vi "Hadamard vs DAQ.vi"() -> ()   [LabVIEW 2023]
uses:
  <vilib>/Utility/miscctls.llb/LVBoundsTypeDef.ctl
  <vilib>/Utility/miscctls.llb/LVRectTypeDef.ctl
panel:
  in  "Plot Area:Size":T1
  out "?":errorcluster
  in  "error in (no error)":errorcluster
  in  "Z Scale.Marker Values[]":cluster{dbl, u32}[](array[cluster])=[{0.0, 0}, {100.0, 16777215}]
  out "Delay":i32=20
  out "Intensity Graph":dbl[][](graph)=[[0.0, 1.0, 0.0, 1.0, 1.0, 0.0, 1.0, 0.0, 0.0, 1.0, 0.0, 1.0, 1.0, 0.0, 1.0, 0.0], [0.0, 1.0, 0.0, 1.0, 1.0, 0.0, 1.0, 0.0, 0.0, 1.0, 0.0, 1.0, 1.0, 0.0, 1.0, 0.0], [1.0, 0.0, 1.0, 0.0, 0.0, 1.0, 0.0, 1.0, 1.0, 0.0, 1.0, 0.0, 0.0, 1.0, 0.0, 1.0], [1.0, 0.0, 1.0, 0.0, 0.0, 1.0, 0.0, 1.0, 1.0, 0.0, 1.0, 0.0, 0.0, 1.0, 0.0, 1.0], [0.0, 1.0, 0.0, 1.0, 1.0, 0.0, 1.0, 0.0, 0.0, 1.0, 0.0, 1.0, 1.0, 0.0, 1.0, 0.0], [0.0, 1.0, 0.0, 1.0, 1.0, 0.0, 1.0, 0.0, 0.0, 1.0, 0.0, 1.0, 1.0, 0.0, 1.0, 0.0], [1.0, 0.0, 1.0, 0.0, 0.0, 1.0, 0.0, 1.0, 1.0, 0.0, 1.0, 0.0, 0.0, 1.0, 0.0, 1.0], [1.0, 0.0, 1.0, 0.0, 0.0, 1.0, 0.0, 1.0, 1.0, 0.0, 1.0, 0.0, 0.0, 1.0, 0.0, 1.0], [0.0, 1.0, 0.0, 1.0, 1.0, 0.0, 1.0, 0.0, 0.0, 1.0, 0.0, 1.0, 1.0, 0.0, 1.0, 0.0], [0.0, 1.0, 0.0, 1.0, 1.0, 0.0, 1.0, 0.0, 0.0, 1.0, 0.0, 1.0, 1.0, 0.0, 1.0, 0.0], [1.0, 0.0, 1.0, 0.0, 0.0, 1.0, 0.0, 1.0, 1.0, 0.0, 1.0, 0.0, 0.0, 1.0, 0.0, 1.0], [1.0, 0.0, 1.0, 0.0, 0.0, 1.0, 0.0, 1.0, 1.0, 0.0, 1.0, 0.0, 0.0, 1.0, 0.0, 1.0], [0.0, 1.0, 0.0, 1.0, 1.0, 0.0, 1.0, 0.0, 0.0, 1.0, 0.0, 1.0, 1.0, 0.0, 1.0, 0.0], [0.0, 1.0, 0.0, 1.0, 1.0, 0.0, 1.0, 0.0, 0.0, 1.0, 0.0, 1.0, 1.0, 0.0, 1.0, 0.0], [1.0, 0.0, 1.0, 0.0, 0.0, 1.0, 0.0, 1.0, 1.0, 0.0, 1.0, 0.0, 0.0, 1.0, 0.0, 1.0], [1.0, 0.0, 1.0, 0.0, 0.0, 1.0, 0.0, 1.0, 1.0, 0.0, 1.0, 0.0, 0.0, 1.0, 0.0, 1.0]]
  out "N":i32=16
  in  "stop":bool
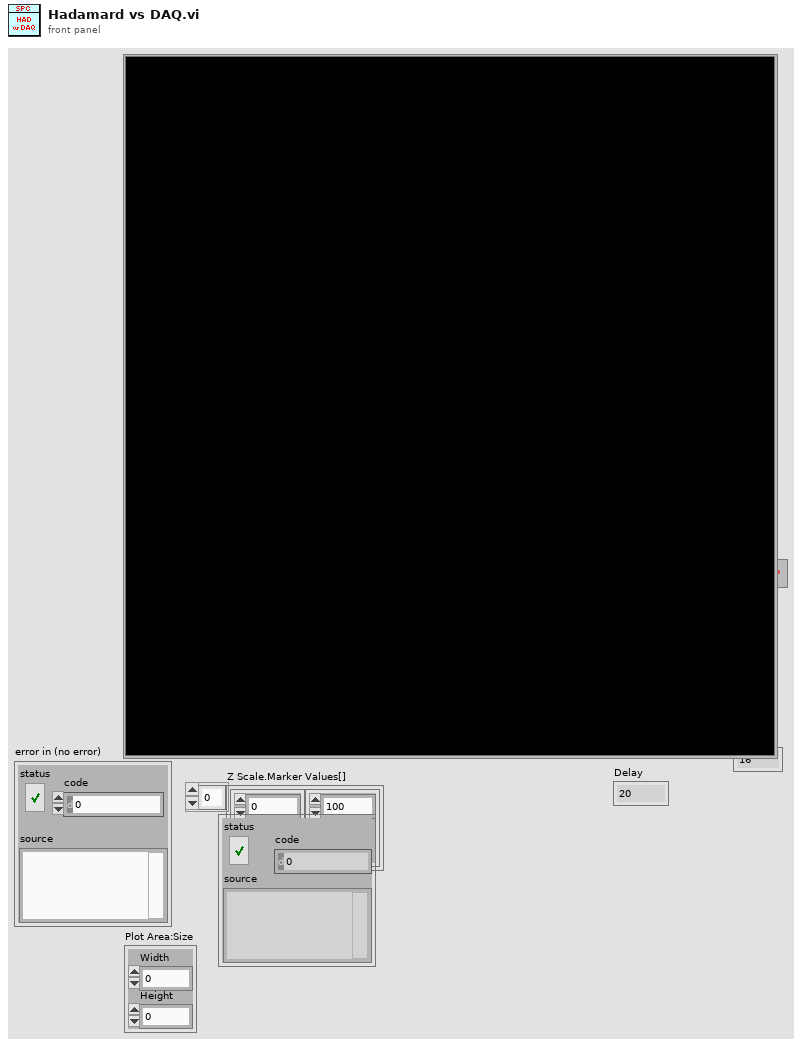
[diagram p1: front panel]
types:
  T1 = typedef "LVBoundsTypeDef.ctl" = cluster{"Width":u32, "Height":u32}
  T2 = typedef "LVRectTypeDef.ctl" = cluster{"Left":i16, "Top":i16, "Right":i16, "Bottom":i16}
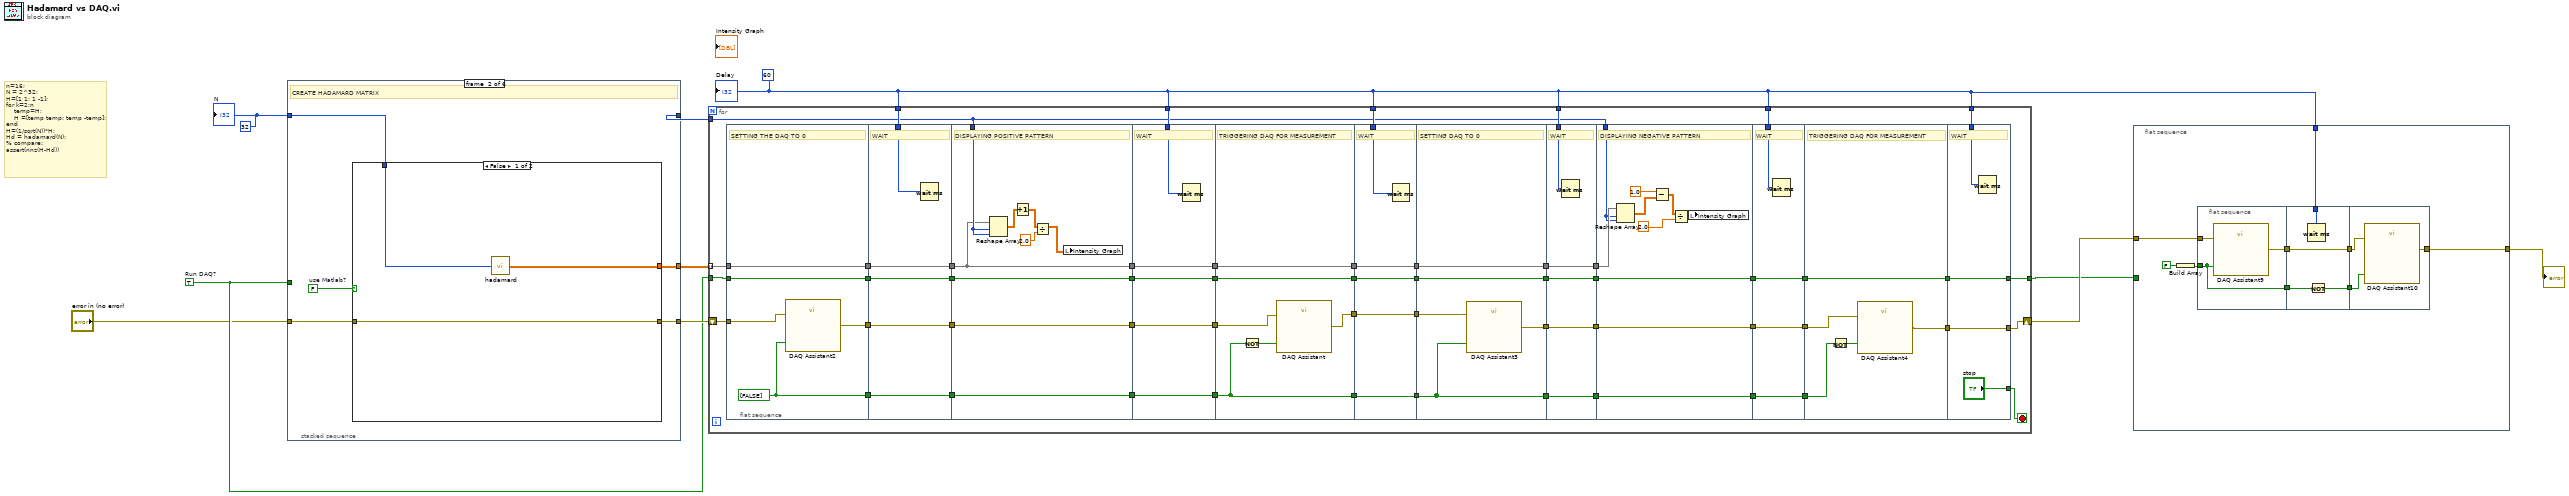
[diagram p0: block diagram]
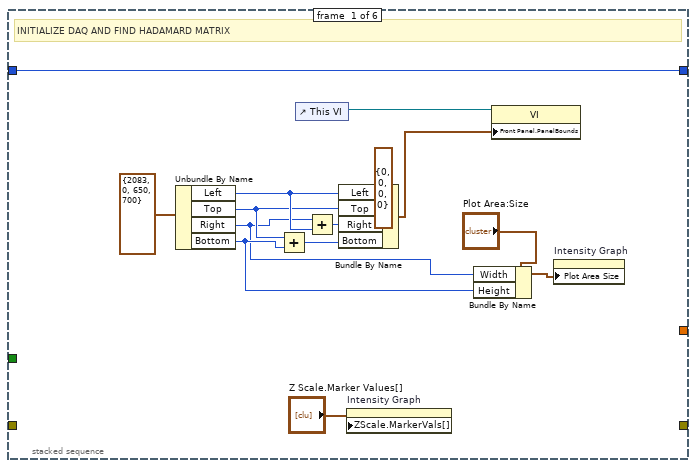
[diagram p2: hidden frame]
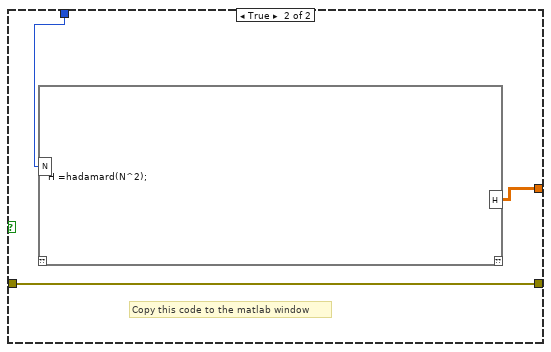
[diagram p3: hidden frame]
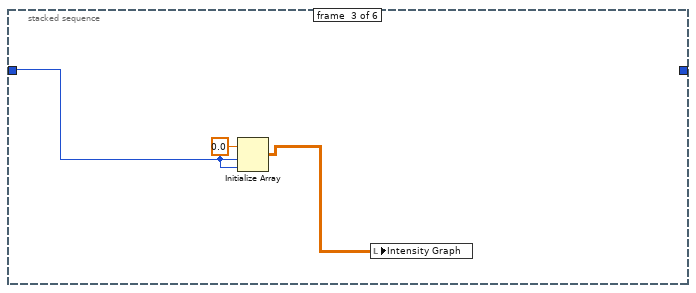
[diagram p4: hidden frame]
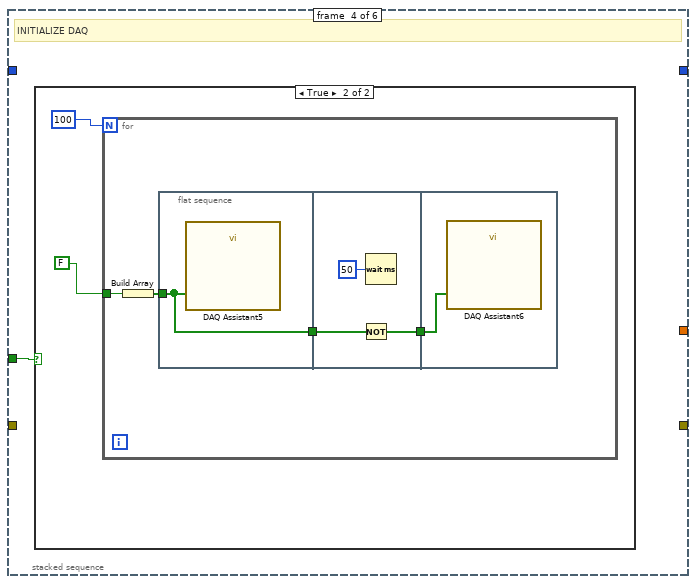
[diagram p5: hidden frame]
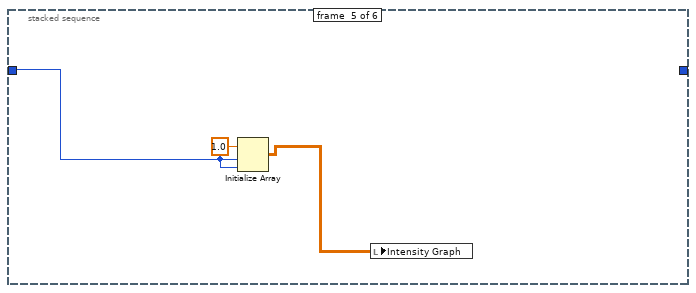
[diagram p7: hidden frame]
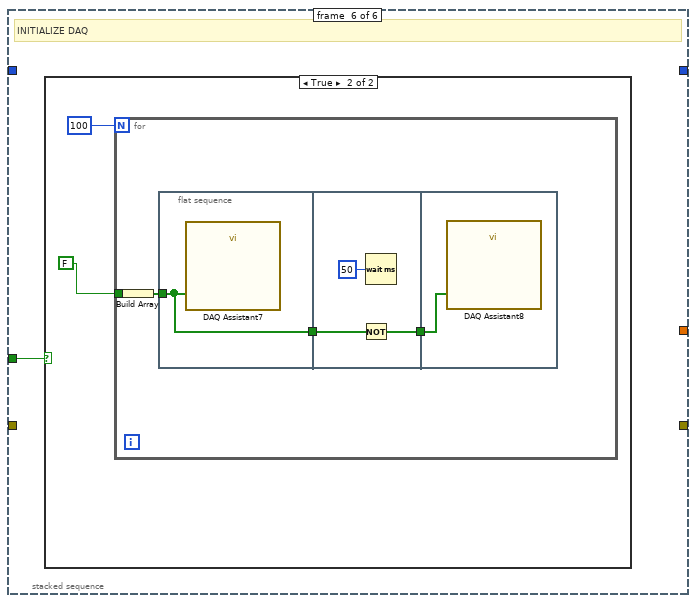
[diagram p8: hidden frame]
diagram:
  w4 = TRUE  # Run DAQ?
  w3 = 60 ("Delay")
  w7 = 32 ("N")
  # "n=16;\nN = 2^32;\nH=[1 1; 1 -1];\nfor k=2:n\n    temp=H;\n    H =[temp temp; temp -temp];\nend\nH=(1/sqrt(N))*H;\nHd = hadamard(N);\n% compare:\nassert(nnz(H-Hd))"
  n1 = stacked-sequence {
    tunnel: [_ w25 _ _ _ _] -> w9
    tunnel: w7 -> [w24 w28 w38 _ w53 _]
    tunnel: [w24 _ _ _ _ _] -> w8
    tunnel: [_ w27 _ _ _ _] -> w10
    tunnel: w4 -> [_ _ _ w39 _ w54]
    tunnel: "error in (no error)" -> [_ w26 _ _ _ _]
    frame #0 {
      # "INITIALIZE DAQ AND FIND HADAMARD MATRIX"
      n2 = Unbundle By Name(T2 {"Left"=2083, "Top"=0, "Right"=650, "Bottom"=700} ("Front Panel Window:Panel Bounds")) -> ("Left"=w20:i16, "Top"=w12:i16, "Right"=w11:i16, "Bottom"=w13:i16)
      n3 = Add(x=w12, y=w13) -> (x+y=w17:i16)
      n4 = control-ref of="This VI"() -> (w22:refnum<vi>)
      n5 = Add(x=w11, y=w20) -> (x+y=w19:i16)
      n6 = Bundle By Name(cluster=T2 {"Left"=0, "Top"=0, "Right"=0, "Bottom"=0} ("output cluster"), "Left"=w20, "Top"=w12, "Right"=w19, "Bottom"=w17) -> (w18:T2)
      n7 = property on="Intensity Graph" class="IntGraph (strict)"("ZScale.MarkerVals[]"="Z Scale.Marker Values[]") -> ()  [unwired: 2 in, 2 out]
      n8 = Bundle By Name(cluster="Plot Area:Size", "Width"=w11, "Height"=w13) -> (w14:T1)
      n9 = property class="VI"(reference=w22, "Front Panel.PanelBounds"=w18) -> ()  [unwired: 1 in, 2 out]
      n10 = property on="Intensity Graph" class="IntGraph (strict)"("Plot Area Size"=w14) -> ()  [unwired: 2 in, 2 out]
    }
    frame #1 {
      w29 = FALSE  # use Matlab?
      # "CREATE HADAMARD MATRIX"
      n11 = case shown="False" w29 {
        tunnel: w28 -> [w32 w34]
        tunnel: [w31 w33] -> w25
        tunnel: [w30 w35] -> w27
        tunnel: w26 -> [w30 w35]
        frame False {
          n12 = call "hadamard.vi"("N"=w32) -> ("Intensity Graph"=w31:dbl[][])
        }
        frame True {
          # "Copy this code to the matlab window"
          n13 = script code="H =hadamard(N^2);"("N"=w34) -> ("H"=w33:dbl[][])  [unwired: 1 in, 1 out]
        }
      }
    }
    frame #2 {
      n14 = Initialize Array(0.0 ("element"), w38, w38) -> (w37:dbl[][])
      n15 = local write "Intensity Graph"(w37) -> ()
    }
    frame #3 {
      # "INITIALIZE DAQ"
      n16 = case shown="True" w39 {
        frame False {
        }
        frame True {
          n17 = for {
            N: 100 -> [_]
            tunnel: FALSE -> [w44]
            n18 = Build Array(w44) -> (w45:bool[])
            n19 = flat-sequence {
              tunnel: w45 -> [w46]
              tunnel: [w46] -> w42
              tunnel: [w47] -> w43
              tunnel: w42 -> [w48]
              tunnel: w43 -> [w50]
              frame #0 {
                n20 = call "DAQ Assistant5"("data"=w46) -> ()  [unwired: 17 in, 2 out]
              }
              frame #1 {
                n21 = Not(x=w48) -> (.not. x?=w47:bool[])
                n22 = Wait (ms)(milliseconds to wait=u32 50) -> ()  [unwired: 1 out]
              }
              frame #2 {
                n23 = call "DAQ Assistant6"("data"=w50) -> ()  [unwired: 17 in, 2 out]
              }
            }
          }
        }
      }
    }
    frame #4 {
      n24 = Initialize Array(1.0 ("element"), w53, w53) -> (w52:dbl[][])
      n25 = local write "Intensity Graph"(w52) -> ()
    }
    frame #5 {
      # "INITIALIZE DAQ"
      n26 = case shown="True" w54 {
        frame False {
        }
        frame True {
          n27 = for {
            N: 100 -> [_]
            tunnel: FALSE -> [w59]
            n28 = Build Array(w59) -> (w60:bool[])
            n29 = flat-sequence {
              tunnel: w60 -> [w61]
              tunnel: [w61] -> w57
              tunnel: [w62] -> w58
              tunnel: w57 -> [w63]
              tunnel: w58 -> [w65]
              frame #0 {
                n30 = call "DAQ Assistant7"("data"=w61) -> ()  [unwired: 17 in, 2 out]
              }
              frame #1 {
                n31 = Not(x=w63) -> (.not. x?=w62:bool[])
                n32 = Wait (ms)(milliseconds to wait=u32 50) -> ()  [unwired: 1 out]
              }
              frame #2 {
                n33 = call "DAQ Assistant8"("data"=w65) -> ()  [unwired: 17 in, 2 out]
              }
            }
          }
        }
      }
    }
  }
  n34 = for {
    tunnel: w9 -> [w118] mode=indexing
    tunnel: w3 -> [w111]
    tunnel: w3 -> [w110]
    tunnel: w3 -> [w109]
    tunnel: w3 -> [w100]
    tunnel: w3 -> [w99]
    tunnel: w3 -> [w94]
    shift-right: [w92] -> w6
    shift-left: w10 -> [w80]
    tunnel: w8 -> [w79]
    tunnel: w4 -> [w78]
    tunnel: [w66] -> w2
    stop <- w93 stop-if-true
    n35 = flat-sequence {
      tunnel: w118 -> [w123]
      tunnel: [w123] -> w116
      tunnel: [w122] -> w112
      tunnel: [w121] -> w84
      tunnel: w80 -> [w120]
      tunnel: w78 -> [w119]
      tunnel: [w119] -> w74
      tunnel: [w128] -> w117
      tunnel: w116 -> [w128]
      tunnel: [w127] -> w113
      tunnel: w112 -> [w127]
      tunnel: w111 -> [w126]
      tunnel: w84 -> [w125]
      tunnel: [w125] -> w83
      tunnel: [w124] -> w75
      tunnel: w74 -> [w124]
      tunnel: w117 -> [w130]
      tunnel: w79 -> [w137]
      tunnel: [w136] -> w114
      tunnel: w113 -> [w136]
      tunnel: [w130] -> w106
      tunnel: w83 -> [w133]
      tunnel: [w133] -> w82
      tunnel: [w129] -> w76
      tunnel: w75 -> [w129]
      tunnel: [w142] -> w115
      tunnel: w114 -> [w142]
      tunnel: w110 -> [w141]
      tunnel: [w140] -> w107
      tunnel: w106 -> [w140]
      tunnel: w82 -> [w139]
      tunnel: [w139] -> w81
      tunnel: [w138] -> w77
      tunnel: w76 -> [w138]
      tunnel: w115 -> [w147]
      tunnel: [w148] -> w108
      tunnel: w107 -> [w148]
      tunnel: [w147] -> w103
      tunnel: [w146] -> w86
      tunnel: w81 -> [w145]
      tunnel: w77 -> [w144]
      tunnel: [w144] -> w72
      tunnel: w109 -> [w153]
      tunnel: [w152] -> w105
      tunnel: w108 -> [w152]
      tunnel: [w151] -> w104
      tunnel: w103 -> [w151]
      tunnel: w86 -> [w150]
      tunnel: [w150] -> w85
      tunnel: [w149] -> w73
      tunnel: w72 -> [w149]
      tunnel: w105 -> [w158]
      tunnel: [w158] -> w102
      tunnel: w104 -> [w157]
      tunnel: [w157] -> w95
      tunnel: [w156] -> w90
      tunnel: w85 -> [w155]
      tunnel: w73 -> [w154]
      tunnel: [w154] -> w67
      tunnel: w102 -> [w163]
      tunnel: [w163] -> w101
      tunnel: w100 -> [w162]
      tunnel: [w161] -> w96
      tunnel: w95 -> [w161]
      tunnel: w90 -> [w160]
      tunnel: [w160] -> w89
      tunnel: [w159] -> w68
      tunnel: w67 -> [w159]
      tunnel: w101 -> [w172]
      tunnel: w79 -> [w171]
      tunnel: [w169] -> w97
      tunnel: w96 -> [w169]
      tunnel: w89 -> [w168]
      tunnel: [w168] -> w88
      tunnel: [w164] -> w69
      tunnel: w68 -> [w164]
      tunnel: w99 -> [w177]
      tunnel: [w176] -> w98
      tunnel: w97 -> [w176]
      tunnel: w88 -> [w175]
      tunnel: [w175] -> w87
      tunnel: [w174] -> w70
      tunnel: w69 -> [w174]
      tunnel: w98 -> [w182]
      tunnel: [w181] -> w91
      tunnel: w87 -> [w178]
      tunnel: [w180] -> w71
      tunnel: w70 -> [w180]
      tunnel: w94 -> [w186]
      tunnel: ["stop"] -> w93
      tunnel: [w184] -> w92
      tunnel: w91 -> [w184]
      tunnel: [w183] -> w66
      tunnel: w71 -> [w183]
      frame #0 {
        w122 = bool[] [FALSE] ("data")
        # "SETTING THE DAQ TO 0"
        n36 = call "DAQ Assistant2"("data"=w122, "error in"=w120) -> ("error out"=w121:errorcluster)  [unwired: 16 in, 1 out]
      }
      frame #1 {
        # "WAIT"
        n37 = Wait (ms)(milliseconds to wait=w126) -> ()  [unwired: 1 out]
      }
      frame #2 {
        # "DISPLAYING POSITIVE PATTERN"
        n38 = Reshape Array(w130, w137, w137) -> (w132:dbl[][])
        n39 = Increment(x=w132) -> (x+1=w131:dbl[][])
        n40 = Divide(x=w131, y=2.0) -> (x/y=w134:dbl[][])
        n41 = local write "Intensity Graph"(w134) -> ()
      }
      frame #3 {
        # "WAIT"
        n42 = Wait (ms)(milliseconds to wait=w141) -> ()  [unwired: 1 out]
      }
      frame #4 {
        # "TRIGGERING DAQ FOR MEASUREMENT"
        n43 = Not(x=w147) -> (.not. x?=w143:bool[])
        n44 = call "DAQ Assistant"("data"=w143, "error in"=w145) -> ("error out"=w146:errorcluster)  [unwired: 16 in, 1 out]
      }
      frame #5 {
        # "WAIT"
        n45 = Wait (ms)(milliseconds to wait=w153) -> ()  [unwired: 1 out]
      }
      frame #6 {
        # "SETTING DAQ TO 0"
        n46 = call "DAQ Assistant3"("data"=w157, "error in"=w155) -> ("error out"=w156:errorcluster)  [unwired: 16 in, 1 out]
      }
      frame #7 {
        # "WAIT"
        n47 = Wait (ms)(milliseconds to wait=w162) -> ()  [unwired: 1 out]
      }
      frame #8 {
        # "DISPLAYING NEGATIVE PATTERN"
        n48 = Reshape Array(w172, w171, w171) -> (w166:dbl[][])
        n49 = Subtract(x=1.0, y=w166) -> (x-y=w165:dbl[][])
        n50 = Divide(x=w165, y=2.0) -> (x/y=w170:dbl[][])
        n51 = local write "Intensity Graph"(w170) -> ()
      }
      frame #9 {
        # "WAIT"
        n52 = Wait (ms)(milliseconds to wait=w177) -> ()  [unwired: 1 out]
      }
      frame #10 {
        # "TRIGGERING DAQ FOR MEASUREMENT"
        n53 = Not(x=w182) -> (.not. x?=w179:bool[])
        n54 = call "DAQ Assistant4"("data"=w179, "error in"=w178) -> ("error out"=w181:errorcluster)  [unwired: 16 in, 1 out]
      }
      frame #11 {
        # "WAIT"
        n55 = Wait (ms)(milliseconds to wait=w186) -> ()  [unwired: 1 out]
      }
    }
  }
  n56 = flat-sequence {
    tunnel: w6 -> [w195]
    tunnel: [w194] -> w5
    tunnel: w3 -> [w193]
    tunnel: w2 -> [_]
    frame #0 {
      n57 = Build Array(FALSE) -> (w187:bool[])
      n58 = flat-sequence {
        tunnel: w187 -> [w198]
        tunnel: [w198] -> w192
        tunnel: w195 -> [w197]
        tunnel: [w196] -> w191
        tunnel: [w201] -> w190
        tunnel: w192 -> [w202]
        tunnel: [w200] -> w189
        tunnel: w191 -> [w200]
        tunnel: w193 -> [w199]
        tunnel: w190 -> [w205]
        tunnel: w189 -> [w204]
        tunnel: [w203] -> w194
        frame #0 {
          n59 = call "DAQ Assistant9"("data"=w198, "error in"=w197) -> ("error out"=w196:errorcluster)  [unwired: 16 in, 1 out]
        }
        frame #1 {
          n60 = Wait (ms)(milliseconds to wait=w199) -> ()  [unwired: 1 out]
          n61 = Not(x=w202) -> (.not. x?=w201:bool[])
        }
        frame #2 {
          n62 = call "DAQ Assistant10"("data"=w205, "error in"=w204) -> ("error out"=w203:errorcluster)  [unwired: 16 in, 1 out]
        }
      }
    }
  }
  "N" <- w7
  "Delay" <- w3
  "?" <- w5
